vi "niFPGA Zero Crossing_m.vi"   [LabVIEW 2017]
doc: "Detects zero crossings of an input signal. The data type you wire to <B>input</B> determines the <B>output</B> data type."
uses:
  <vilib>/rvi/Analysis/common/FxpNativeNode/niFpgaFxpNative.xnode
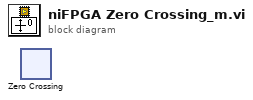
[diagram p0: block diagram]
diagram:
  n1 = xnode ("Zero Crossing")() -> ()  [unwired: 3 in, 1 out]
